vi "Plugin.Get Transceiver Thread.vi"(10 "index":i32, 11 "Plugin in":refnum<class "Plugin.lvclass">) -> (2 "Transceiver Thread":refnum<class "Transceiver Interface.lvclass">, 3 "Plugin out":refnum<class "Plugin.lvclass">)   [LabVIEW 2017, in "DSF Core.lvlib" / "Plugin.lvclass"]
uses:
  Plugin.lvclass
  Interfaces/Transceiver Interface/Transceiver Interface.lvclass
  Plugin.lvclass/Plugin.ctl
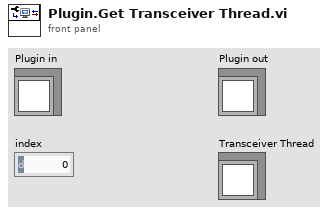
[diagram p1: front panel]
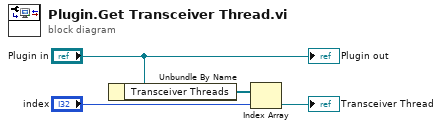
[diagram p0: block diagram]
diagram:
  n1 = Unbundle By Name("Plugin in") -> ("Transceiver Threads"=w3:refnum<class "Transceiver Interface.lvclass">[])
  n2 = Index Array(array=w3, index="index") -> (element=→"Transceiver Thread":refnum<class "Transceiver Interface.lvclass">)
  "Plugin out" <- "Plugin in"
